vi "serial comms L0.vi"(6 "delay before read (ms)":u32=10, 7 "Comms Control":T2(ring), 8 "error IN":errorcluster, 9 "Command String":string="?VW", 10 "Serial Settings":T1={"VISA resource name "="", "baud rate"=8, "data bits"=0, "parity"=enum."Space", "stop bits"=0, "flow control"=0} {"flow control" items=["None"=0, "XON/XOFF"=1, "RTS/CTS"=2, "DTR/DSR"=4]; "stop bits" items=["None"=0, "XON/XOFF"=1, "RTS/CTS"=2, "DTR/DSR"=4]; "baud rate" items=["75"=75, "110"=110, "134"=134, "150"=150, "300"=300, "600"=600, "1200"=1200, "1800"=1800, "2400"=2400, "4800"=4800, "7200"=7200, "9600"=9600, "14400"=14400, "19200"=19200, "28800"=28800, "38400"=38400, "56000"=56000, "57600"=57600, "115200"=115200, "128000"=128000, "230400"=230400]}, 11 "VISA resource name":refnum<visa-resource-name>) -> (0 "Error OUT":errorcluster, 1 "bytes read":u32, 2 "Response":string, 3 "VISA resource name out":refnum<visa-resource-name>, 4 "return count":u32, 5 "output cluster":cluster{bool, i32, bool, i32})   [LabVIEW 2017]
uses:
  Serial - Settings.ctl
  <vilib>/Instr/_visa.llb/VISA Configure Serial Port (Instr).vi
panel:
  out "Read bytes failed":bool
  out "Bytes at port failed":bool
  out "Read bytes loop itr":i32
  out "Bytes at port loop itr":i32
  out "VISA resource out":refnum<visa-resource-name>
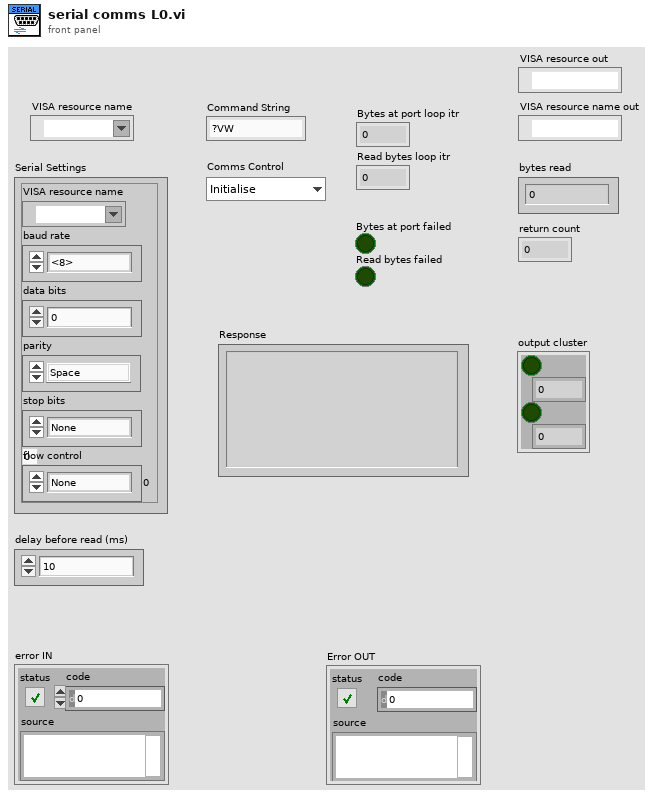
[diagram p1: front panel]
types:
  T1 = typedef "Serial - Settings.ctl" = cluster{"VISA resource name ":refnum<visa-resource-name>, "baud rate":u32, "data bits":u16, "parity":enum16{"None", "Odd", "Even", "Mark", "Space"}, "stop bits":u16, "flow control":u16}
  T2 = enum16{"Initialise", "Read Handle", "Command & Query", "Close"}
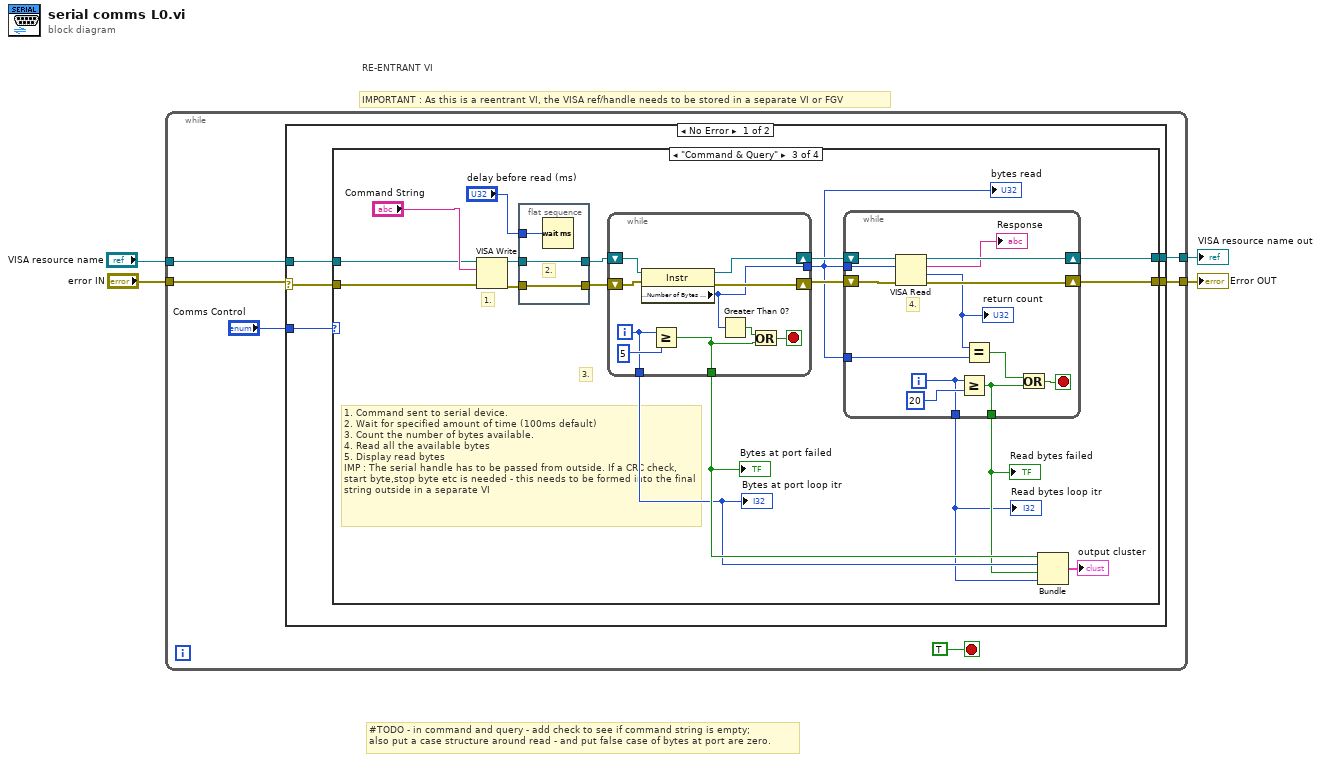
[diagram p0: block diagram]
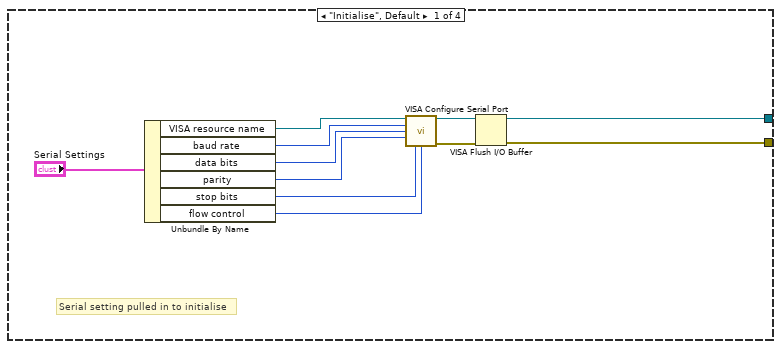
[diagram p2: hidden frame]
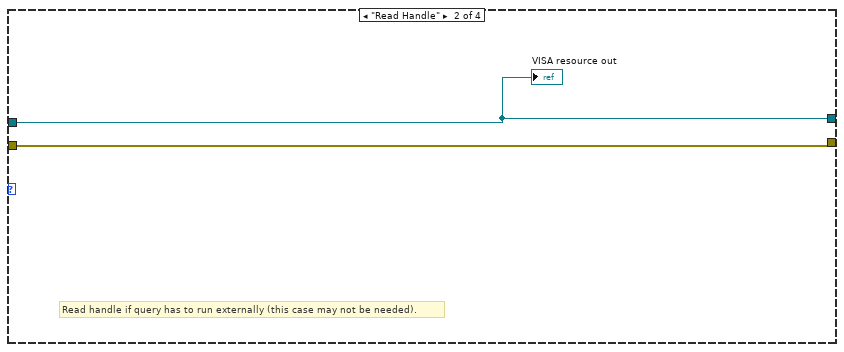
[diagram p3: hidden frame]
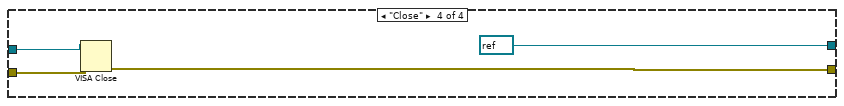
[diagram p4: hidden frame]
diagram:
  # "#TODO - in command and query - add check to see if command string is empty;\nalso put a case structure around read - and put false case of bytes at port are zero."
  # "RE-ENTRANT VI"
  # "IMPORTANT : As this is a reentrant VI, the VISA ref/handle needs to be stored in a separate VI or FGV"
  n1 = while {
    tunnel: "error IN" -> [w5]
    tunnel: [w7] -> w3
    tunnel: "VISA resource name" -> [w8]
    tunnel: [w9] -> w2
    stop <- TRUE stop-if-true
    n2 = case shown="No Error" w5 {
      selector: w5 -> [w11 w77]
      tunnel: "Comms Control" -> [w15 _]
      tunnel: [w14 w78] -> w9
      tunnel: w8 -> [w13 w78]
      tunnel: [w12 w77] -> w7
      frame No Error {
        n3 = case shown="\"Command & Query\"" w15 {
          tunnel: [w16 w28 w40 refnum<visa-resource-name> refnum ("VISA resource name out")] -> w14
          tunnel: w13 -> [_ w28 w37 w76]
          tunnel: [w18 w27 w41 w73] -> w12
          tunnel: w11 -> [_ w27 w38 w74]
          frame "Initialise", Default {
            # "Serial setting pulled in to initialise"
            n4 = Unbundle By Name("Serial Settings") -> ("VISA resource name"=w20:refnum<visa-resource-name>, "baud rate"=w22:u32, "data bits"=w23:u16, "parity"=w24:enum16{"None", "Odd", "Even", "Mark", "Space"}, "stop bits"=w25:u16, "flow control"=w26:u16)
            n5 = call-poly "VISA Configure Serial Port"("VISA resource name"=w20, "baud rate (9600)"=w22, "data bits (8)"=w23, "parity (0:none)"=w24, "stop bits (10: 1 bit)"=w25, "flow control (0:none)"=w26) -> ("VISA resource name out"=w17:refnum<visa-resource-name>, "error out"=w19:errorcluster)  [unwired: 3 in, 5 out]
            n6 = VISA Flush I/O Buffer(VISA resource name=w17, error in (no error)=w19) -> (VISA resource name out=w16:refnum<visa-resource-name>, error out=w18:errorcluster)  [unwired: 1 in]
          }
          frame "Read Handle" {
            # "Read handle if query has to run externally (this case may not be needed)."
            "VISA resource out" <- w28
          }
          frame "Command & Query" {
            # "3."
            # "1."
            # "1. Command sent to serial device.\n2. Wait for specified amount of time (100ms default)\n3. Count the number of bytes available.\n4. Read all the available bytes\n5. Display read bytes\nIMP : The serial handle has to be passed from outside. If a CRC check, start byte,stop byte etc is needed - this needs to be formed into the final string outside in a separate VI"
            n7 = VISA Write(VISA resource name=w37, write buffer="Command String", error in (no error)=w38) -> (VISA resource name out=w44:refnum<visa-resource-name>, error out=w42:errorcluster)  [unwired: 1 out]
            n8 = flat-sequence {
              tunnel: w42 -> [w71]
              tunnel: [w71] -> w43
              tunnel: w44 -> [w70]
              tunnel: [w70] -> w45
              tunnel: "delay before read (ms)" -> [w72]
              frame #0 {
                # "2."
                n9 = Wait (ms)(milliseconds to wait=w72) -> ()  [unwired: 1 out]
              }
            }
            n10 = while {
              tunnel: [w65] -> w34
              shift-right: [w66] -> w35
              shift-left: w45 -> [w69]
              shift-right: [w67] -> w36
              shift-left: w43 -> [w68]
              tunnel: [w61] -> w32
              tunnel: [w60] -> w33
              i -> [w61]
              stop <- w62 stop-if-true
              n11 = property class="Instr"(reference=w69, error in=w68) -> (reference out=w66:refnum<visa-resource-name>, error out=w67:errorcluster, "Serial Settings:Number of Bytes at Serial Port"=w65:u32)
              n12 = Greater Or Equal?(x=w61, y=5) -> (x >= y?=w60:bool)
              n13 = Greater Than 0?(x=w65) -> (x > 0?=w63:bool)
              n14 = Or(x=w63, y=w60) -> (x .or. y?=w62:bool)
            }
            "bytes read" <- w34
            "Bytes at port loop itr" <- w32
            "Bytes at port failed" <- w33
            n15 = while {
              tunnel: w34 -> [w56]
              shift-right: [w59] -> w41
              shift-left: w36 -> [w55]
              shift-right: [w58] -> w40
              shift-left: w35 -> [w54]
              tunnel: w34 -> [w52]
              tunnel: [w48] -> w30
              tunnel: [w47] -> w31
              i -> [w48]
              stop <- w49 stop-if-true
              # "4."
              n16 = VISA Read(VISA resource name=w54, byte count=w56, error in (no error)=w55) -> (VISA resource name out=w58:refnum<visa-resource-name>, read buffer=→"Response":string, return count=w53:u32, error out=w59:errorcluster)
              "return count" <- w53
              n17 = Greater Or Equal?(x=w48, y=20) -> (x >= y?=w47:bool)
              n18 = Equal?(x=w53, y=w52) -> (x = y?=w50:bool)
              n19 = Or(x=w50, y=w47) -> (x .or. y?=w49:bool)
            }
            "Read bytes loop itr" <- w30
            "Read bytes failed" <- w31
            n20 = Bundle(w33, w32, w31, w30) -> (→"output cluster":cluster{bool, i32, bool, i32})  [unwired: 1 in]
          }
          frame "Close" {
            n21 = VISA Close(VISA resource name=w76, error in (no error)=w74) -> (error out=w73:errorcluster)
          }
        }
      }
      frame Error {
      }
    }
  }
  "Error OUT" <- w3
  "VISA resource name out" <- w2
